vi "BuildPosString.vi"(7 "Z val":dbl, 8 "error in (no error)":errorcluster, 9 "XY":cluster{"X":dbl, "Y":dbl}, 10 "Y graph pixels":i32, 11 "X graph pixels":i32) -> (0 "error out":errorcluster, 3 "String":string)   [LabVIEW 2023]
doc: "Builds position String from X,Y Values, XPx,YPx and Z Value."
uses:
  StringFormatGlobals.vi
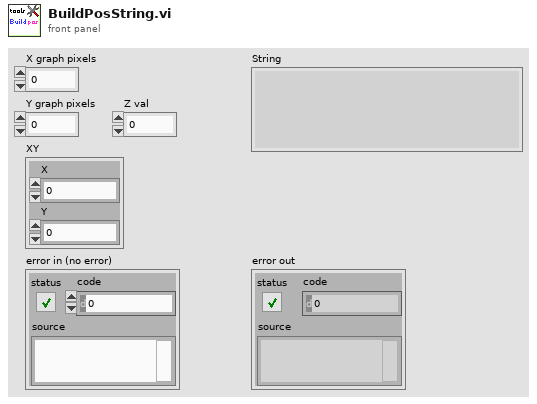
[diagram p1: front panel]
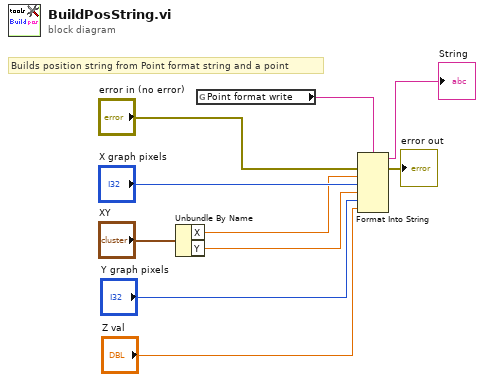
[diagram p0: block diagram]
diagram:
  # "Builds position string from Point format string and a point"
  n1 = Unbundle By Name("XY") -> ("X"=w5:dbl, "Y"=w6:dbl)
  n2 = global read "StringFormatGlobals.vi" "Point format write"() -> (w1:string)
  n3 = Format Into String(format string=w1, error in="error in (no error)", w5, "X graph pixels", w6, "Y graph pixels", "Z val") -> (resulting string=→"String":string, error out=→"error out":errorcluster)  [unwired: 1 in]
